vi "Main6.vi"() -> ()   [LabVIEW 2014]
doc: "The myRIO Project template acquires acceleration data from the onboard accelerometer and displays the changes of acceleration values in a waveform chart."
uses:
  <vilib>/myRIO/Instrument Drivers/Onboard IO/AI/typedefs/AI Reference.ctl
  <vilib>/myRIO/Common/Instrument Driver Framework/Utilities/typedefs/myRIO Generic Hardware Reference.ctl
  <vilib>/myRIO/Common/Instrument Driver Framework/Utilities/typedefs/Hardware Version Enum.ctl
  <vilib>/myRIO/Common/Instrument Driver Framework/Utilities/typedefs/myRIO v1.0 Reference.ctl
  <vilib>/myRIO/Common/Instrument Driver Framework/Utilities/typedefs/Generic FPGA Reference.ctl
  <vilib>/myRIO/Common/Instrument Driver Framework/myRIO v1.0/AI/typedefs/AI Channels List.ctl
  <vilib>/myRIO/Common/Instrument Driver Framework/myRIO v1.0/AI/typedefs/AI Channels Enum.ctl
  <vilib>/myRIO/Common/Instrument Driver Framework/Utilities/typedefs/Analog Scaling Constants List.ctl
  <vilib>/myRIO/Common/Instrument Driver Framework/Utilities/typedefs/Analog Scaling Constants.ctl
  <vilib>/userdefined/High Color/nirio_resource_hc.ctl
  <vilib>/myRIO/Instrument Drivers/Onboard IO/DIO/typedefs/DIO Reference.ctl
  <vilib>/myRIO/Common/Instrument Driver Framework/myRIO v1.0/DIO/typedefs/DIO Channels List.ctl
  <vilib>/myRIO/Common/Instrument Driver Framework/myRIO v1.0/DIO/typedefs/DIO Channels Enum.ctl
  <vilib>/myRIO/Common/Instrument Driver Framework/Utilities/vis/Is FPGA Ref Available.vi
  <vilib>/myRIO/Common/Instrument Driver Framework/myRIO v1.0/AI/vis/myRIO v1.1 Open AI.vi
  <vilib>/myRIO/Instrument Drivers/Onboard IO/AI/vis/Read.vi
  <vilib>/myRIO/Common/Instrument Driver Framework/myRIO v1.0/DIO/vis/myRIO v1.1 Open DIO.vi
  <vilib>/myRIO/Instrument Drivers/Onboard IO/DIO/vis/Write.vi
  <vilib>/myRIO/Common/Instrument Driver Framework/Utilities/vis/Validate Channels.vi
  <vilib>/myRIO/Common/Instrument Driver Framework/myRIO v1.0/AI/vis/myRIO v1.0 Reserve AI.vi
  <vilib>/myRIO/Common/Instrument Driver Framework/myRIO v1.0/DIO/vis/myRIO v1.0 Reserve DIO.vi
  <vilib>/myRIO/Common/Instrument Driver Framework/myRIO v1.0/AI/vis/myRIO v1.0 Build MUX Configuration AI.vi
  <vilib>/myRIO/Common/Instrument Driver Framework/myRIO v1.0/Resource Manager/vis/myRIO v1.0 Reserve Channel List.vi
  <vilib>/myRIO/Common/Instrument Driver Framework/myRIO v1.0/DIO/vis/myRIO v1.0 Build MUX Configuration DIO.vi
  <vilib>/myRIO/Common/Instrument Driver Framework/myRIO v1.0/Resource Manager/vis/myRIO v1.0 Reserve Channel.vi
  <vilib>/myRIO/Common/Instrument Driver Framework/myRIO v1.0/Resource Manager/vis/myRIO v1.0 Unreserve Channel.vi
  <vilib>/myRIO/Common/Instrument Driver Framework/myRIO v1.0/Resource Manager/vis/myRIO v1.0 Create Configuration List.vi
  <vilib>/myRIO/Common/Instrument Driver Framework/myRIO v1.0/Resource Manager/vis/myRIO v1.0 Build Mutex Name.vi
  <vilib>/Utility/VariantDataType/GetNumericInfo.vi
  <vilib>/Utility/error.llb/Error Cluster From Error Code.vi
  <vilib>/myRIO/Common/Instrument Driver Framework/myRIO v1.0/myRIO v1.1 Open.vi
  <vilib>/myRIO/Common/Instrument Driver Framework/myRIO v1.0/AI/vis/myRIO v1.0 Get Scaling Constants AI.vi
  <vilib>/myRIO/Common/Instrument Driver Framework/Utilities/vis/IO Manager.vi
  <vilib>/myRIO/Common/Instrument Driver Framework/Utilities/vis/Configuration Manager.vi
  <vilib>/myRIO/Common/Instrument Driver Framework/myRIO v1.0/myRIO v1.0 Close.vi
  <vilib>/myRIO/Common/Instrument Driver Framework/myRIO v1.0/AI/vis/myRIO v1.0 Read AI.vi
  <vilib>/myRIO/Common/Instrument Driver Framework/myRIO v1.0/Resource Manager/vis/myRIO v1.0 Configure IO.vi
  <vilib>/myRIO/Common/Instrument Driver Framework/myRIO v1.0/DIO/vis/myRIO v1.0 Write DIO.vi
  <vilib>/myRIO/Express VI/Onboard IO/AI/AI Express VI.xnode
  <vilib>/myRIO/Instrument Drivers/Onboard IO/AI/vis/myRIO AI Open.xnode
  <vilib>/myRIO/Express VI/Onboard Devices/LED/LED Express VI.xnode
  <vilib>/myRIO/Instrument Drivers/Onboard IO/DIO/vis/myRIO DIO Open.xnode
  <vilib>/vision/driver/NI_Vision_Acquisition_Software.lvlib
  <vilib>/vision/NI_Vision_Development_Module.lvlib
  <vilib>/myRIO/Instrument Drivers/Onboard IO/AI/AI.lvlib
  <vilib>/myRIO/Instrument Drivers/Onboard IO/DIO/DIO.lvlib
panel:
  in  "숫자형":dbl
  in  "탭 컨트롤":enum32{"볼링핀 0", "배경 1", "녹색핀 2"}(tab)
  in  "Blue or Luminance":cluster{i32, i32}(slide)={170, 255} scale=0.0..255.0
  in  "Green or Saturation":cluster{i32, i32}(slide)={0, 90} scale=0.0..255.0
  in  "Red or Hue":cluster{i32, i32}(slide)={0, 255} scale=0.0..255.0
  in  "Blue or Luminance 2":cluster{i32, i32}(slide)={0, 145} scale=0.0..255.0
  in  "Green or Saturation 2":cluster{i32, i32}(slide)={1, 41} scale=0.0..255.0
  in  "Red or Hue 2":cluster{i32, i32}(slide)={0, 255} scale=0.0..255.0
  in  "Blue or Luminance 3":cluster{i32, i32}(slide)={60, 255} scale=0.0..255.0
  in  "Green or Saturation 3":cluster{i32, i32}(slide)={35, 255} scale=0.0..255.0
  in  "Red or Hue 3":cluster{i32, i32}(slide)={50, 130} scale=0.0..255.0
  in  "Select Servo":string(combo)="Servo 1"
  in  "Controller Daisy Chain Position (1 - 4)":u8=1
  out "x <= y?":bool=TRUE
  out "불리언":bool
  out "x/y":dbl=323.5
  out "Acceleration 4":dbl(graph)=1.2646485669999998
  out "x*y":dbl=4.429408028571429
  out "Acceleration 3":dbl(graph)=4.429408028571429
  out "x-y":dbl=-3.5
  in  "y":dbl=20.0
  out "범위내?":bool=TRUE
  out "웨이브폼 차트 2":dbl(graph)=-0.0
  in  "3":u8=3
  in  "Controller 2":u8=2
  in  "Number of Erosion":i32=2
  in  "Threshold Color Mode":enum32{"RGB", "HSL"}(radio)=enum."HSL"
  out "Image 2":T1(plugin-control)
  in  "Stop 2":bool
  out "Image":T1(plugin-control)
  in  "Camera Name":refnum<k21>="cam3" caption="IMAQdx Session"
  # "Control Motor"
  # "Read Encoder"
  # "흰색 : 0/255"
  # "흰색 : 0/90~140"
  # "흰색 : 160~170/255"
  # "흰색 : 0/255"
  # "흰색 : 0/90"
  # "흰색 : 170/255"
  # "녹색 : 50/130"
  # "녹색 : 35/255"
  # "녹색 : 60/255"
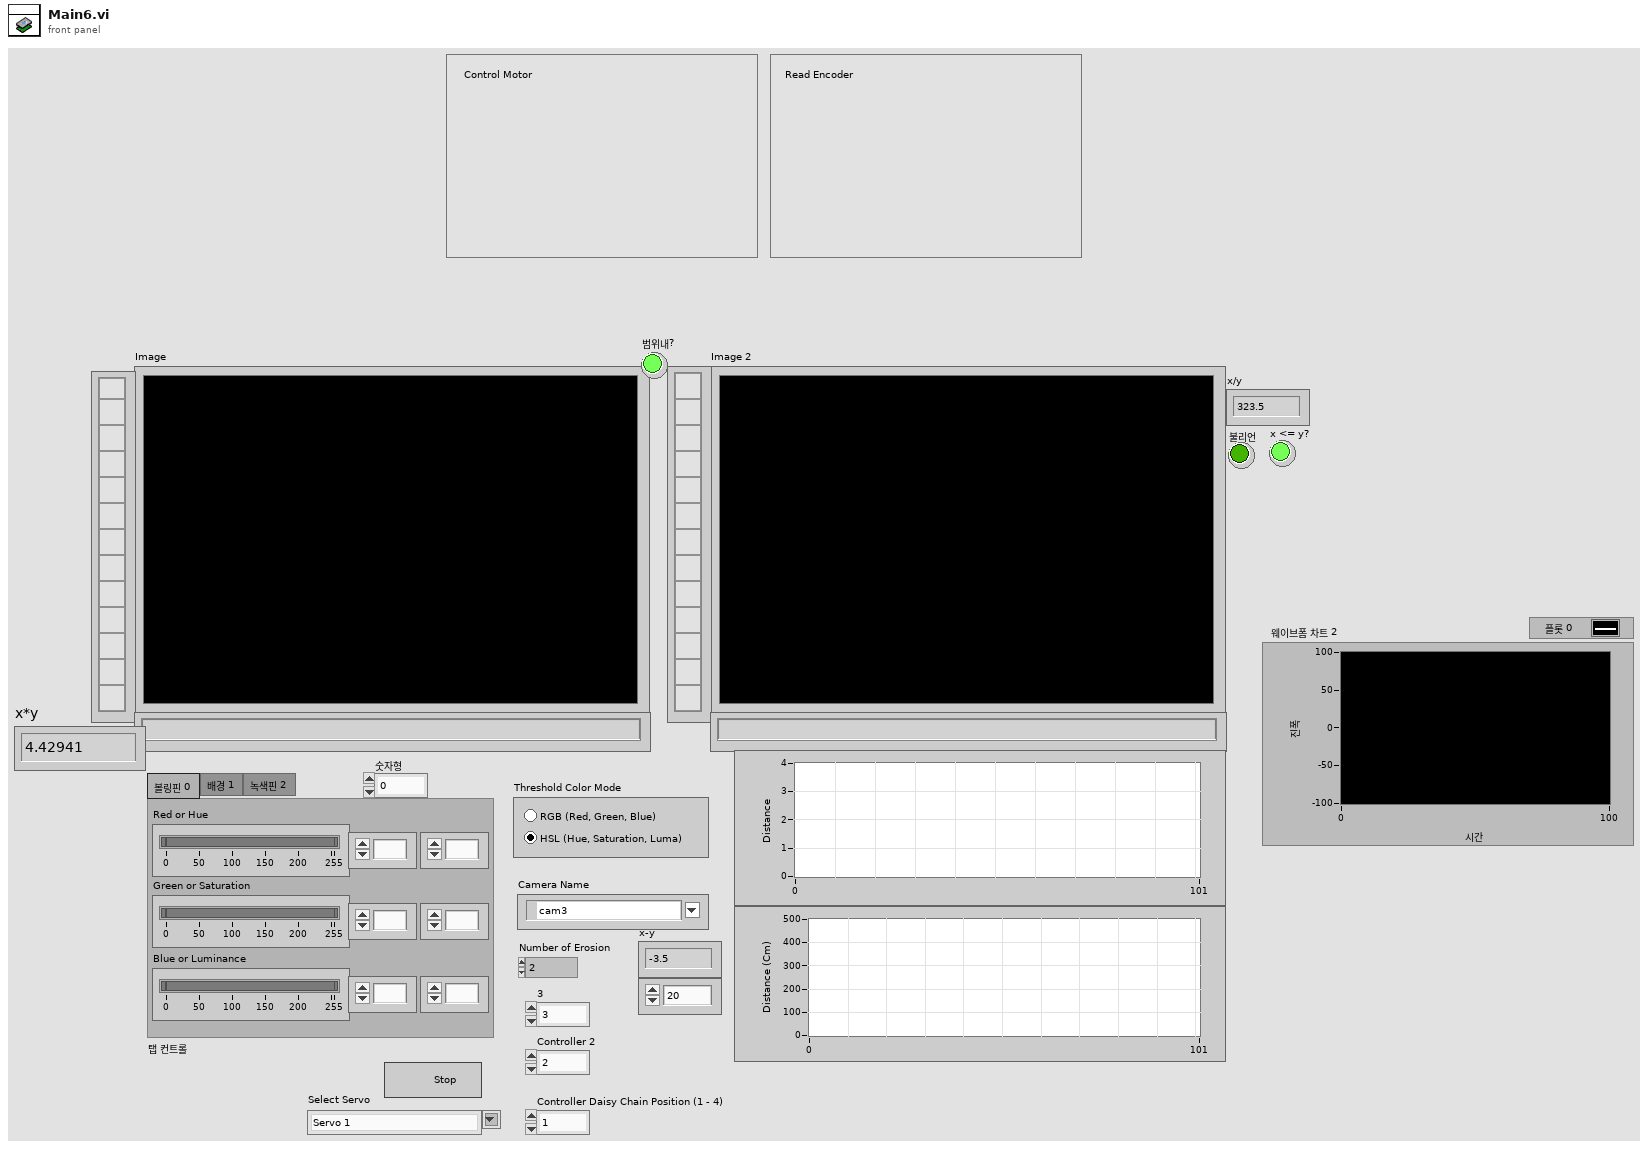
[diagram p1: front panel]
types:
  T1 = typedef "IMAQ Image.ctl" = refnum<image>
  T2 = typedef "DIO.lvlib/DIO Reference.ctl" = cluster{"myRIO Reference":T3, "DIO Channels List":T7}
  T3 = typedef "myRIO Generic Hardware Reference.ctl" = cluster{"myRIO Model":T4, "myRIO Hardware Reference":T5}
  T4 = typedef "Hardware Version Enum.ctl" = enum16{"Unknown", "myRIO-1900", "myRIO-1950"}
  T5 = typedef "myRIO v1.0 Reference.ctl" = cluster{"Generic FPGA Reference":T6, "Allow multiple opens":bool}
  T6 = typedef "Generic FPGA Reference.ctl" = refnum<k20>
  T7 = typedef "DIO Channels List.ctl" = T8[]
  T8 = typedef "DIO Channels Enum.ctl" = enum16{"Not Connected", "C/DIO0", "C/DIO1", "C/DIO2", "C/DIO3", "C/DIO4", "C/DIO5", "C/DIO6", "C/DIO7", "A/DIO0", "A/DIO1", "A/DIO2", "A/DIO3", "A/DIO4", "A/DIO5", "A/DIO6", "A/DIO7", "A/DIO8", "A/DIO9", "A/DIO10", "A/DIO11", "A/DIO12", "A/DIO13", "A/DIO14", "A/DIO15", "B/DIO0", "B/DIO1", "B/DIO2", "B/DIO3", "B/DIO4", "B/DIO5", "B/DIO6", "B/DIO7", "B/DIO8", "B/DIO9", "B/DIO10", "B/DIO11", "B/DIO12", "B/DIO13", "B/DIO14", "B/DIO15", "LED0", "LED1", "LED2", "LED3", "Button0"}
  T9 = typedef "nirio_resource_hc.ctl" = tag
  T10 = typedef "AI.lvlib/AI Reference.ctl" = cluster{"myRIO Reference":T3, "AI Channels List":T11, "AI Scaling Constants List":T13}
  T11 = typedef "AI Channels List.ctl" = T12[]
  T12 = typedef "AI Channels Enum.ctl" = enum16{"Not Connected", "AudioIn/Left", "AudioIn/Right", "C/AI0", "C/AI1", "A/AI0", "A/AI1", "A/AI2", "A/AI3", "B/AI0", "B/AI1", "B/AI2", "B/AI3"}
  T13 = typedef "Analog Scaling Constants List.ctl" = T14[]
  T14 = typedef "Analog Scaling Constants.ctl" = cluster{"LSB Weight (Volts)":dbl, "Offset (Volts)":dbl, "Signed?":bool}
  T15 = typedef "IMAQ Rectangle" = cluster{"Left":i32, "Top":i32, "Right":i32, "Bottom":i32, "Rotation":dbl}
  T16 = typedef "Image Type" = u32
  T17 = typedef "IMAQdx.ctl" = refnum<k21>
  T18 = cluster{"Global Rectangle":i32[], "Contours":cluster{"Contour Type":u32, "ROI Type":u32, "Points":i32[]}[]}
  T19 = cluster{"Area":dbl, "Number of Holes":dbl, "Bounding Rect":cluster{"Left":dbl, "Top":dbl, "Right":dbl, "Bottom":dbl}, "Center of Mass":cluster{"X":dbl, "Y":dbl}, "Orientation":dbl, "Dimensions":cluster{"Width":dbl, "Height":dbl}}[]
  T20 = cluster{"Left":dbl, "Top":dbl, "Right":dbl, "Bottom":dbl}
  T21 = typedef "ROI Descriptor" = cluster{"Global Rectangle":i32[], "Contours":cluster{"ID":enum32{"External", "Internal"}, "Type":u32, "Coordinates":i32[]}[]}
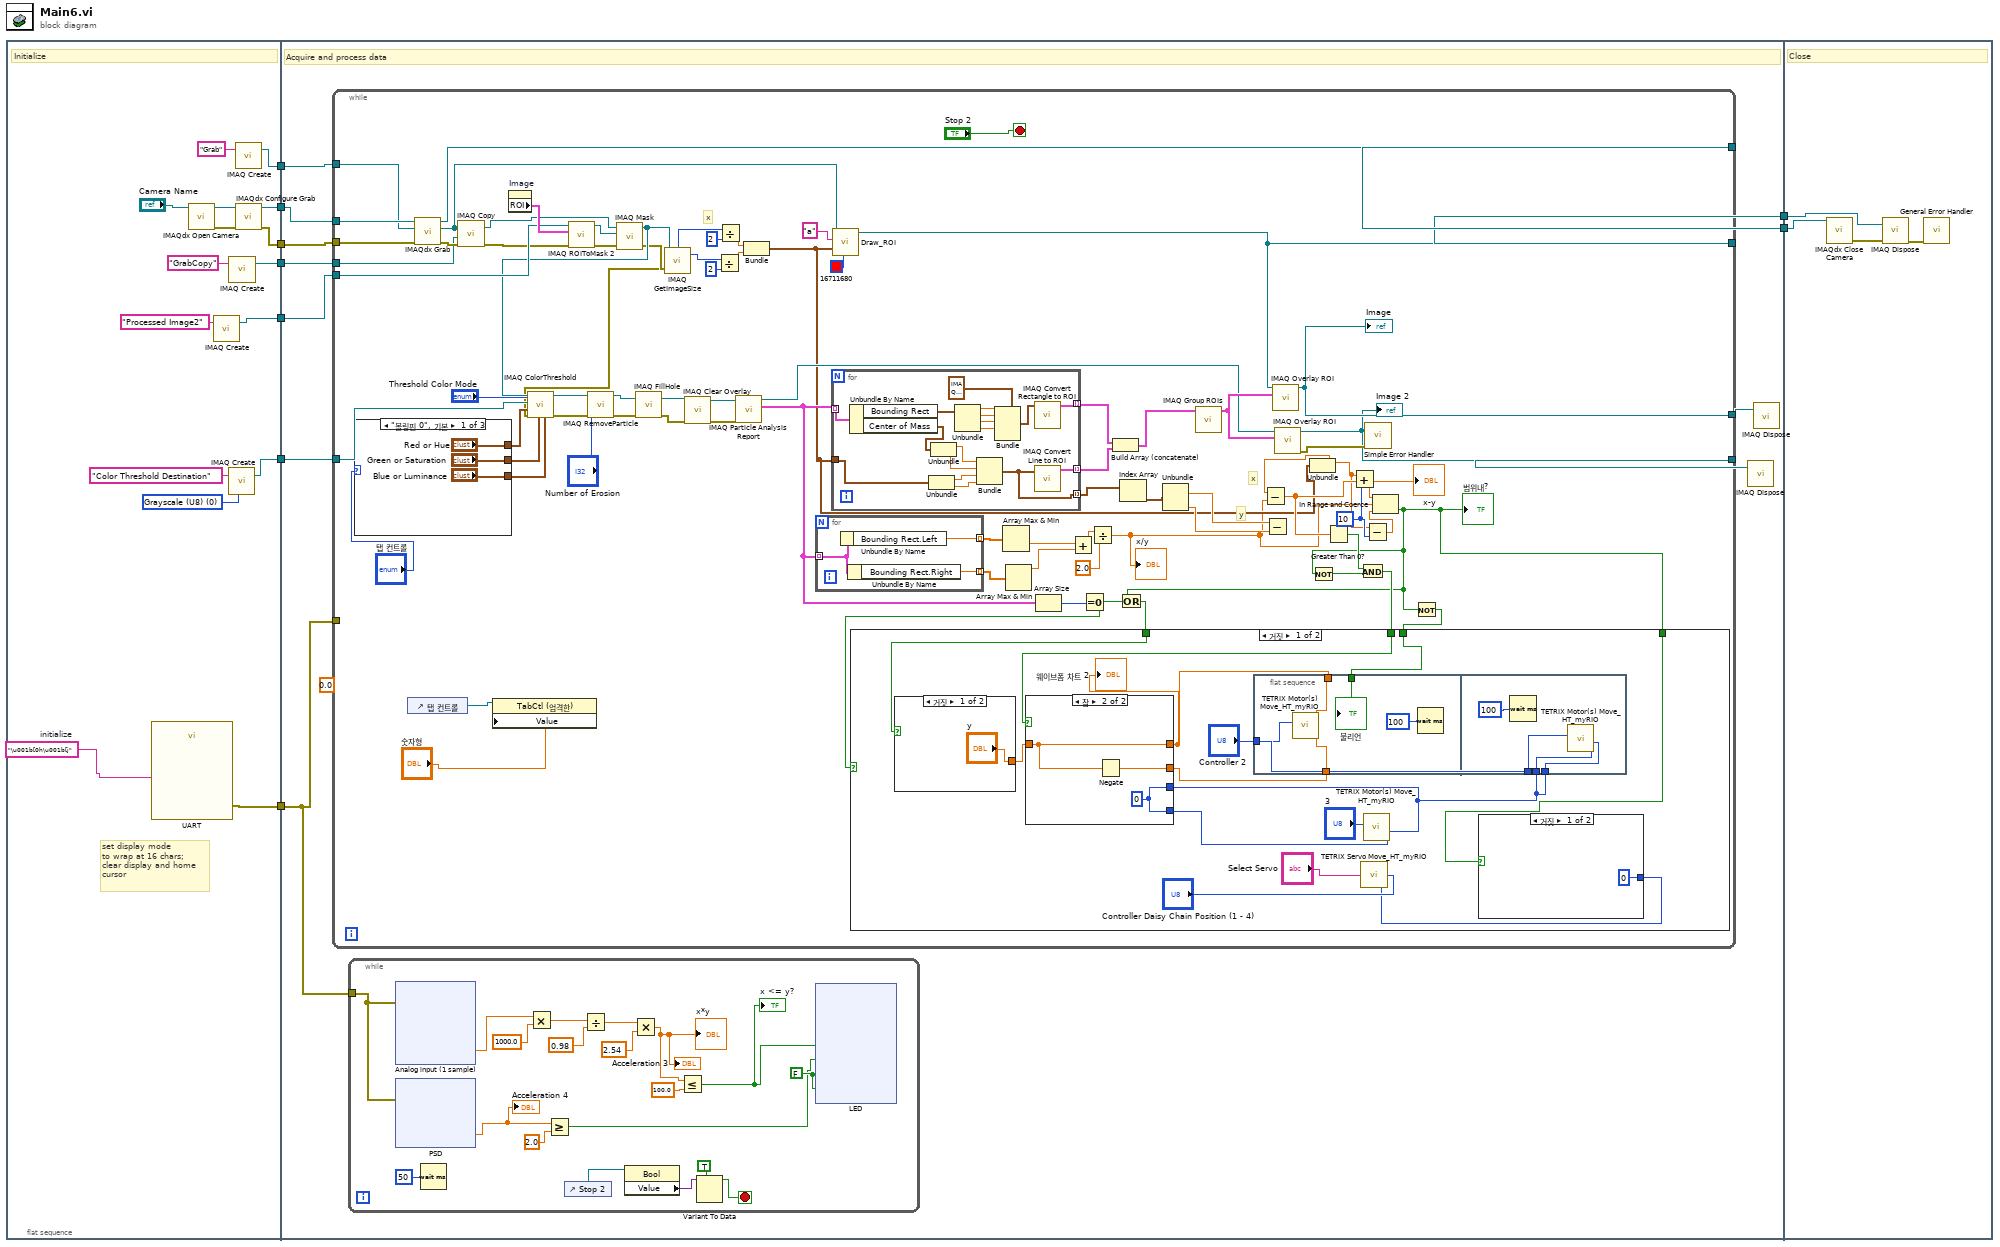
[diagram p0: block diagram]
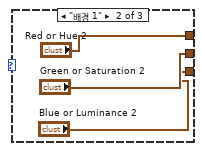
[diagram p2: hidden frame]
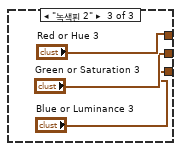
[diagram p3: hidden frame]
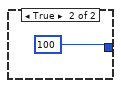
[diagram p4: hidden frame]
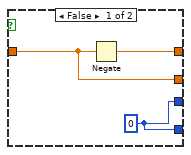
[diagram p5: hidden frame]
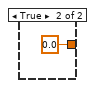
[diagram p6: hidden frame]
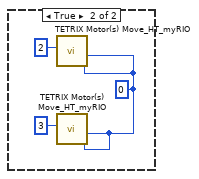
[diagram p7: hidden frame]
diagram:
  n1 = flat-sequence {
    tunnel: [w21] -> w9
    tunnel: [w20] -> w8
    tunnel: [w19] -> w7
    tunnel: [w17] -> w4
    tunnel: [w15] -> w3
    tunnel: [w14] -> w2
    tunnel: [w11] -> w1
    tunnel: w9 -> [w36]
    tunnel: w8 -> [w35]
    tunnel: w7 -> [w34]
    tunnel: [w28] -> w6
    tunnel: [w33] -> w5
    tunnel: w4 -> [w30]
    tunnel: w3 -> [w29]
    tunnel: w2 -> [w26]
    tunnel: w1 -> [w27]
    tunnel: w6 -> [w311]
    tunnel: w5 -> [w310]
    frame #0 {
      w10 = "\u001b[0h\u001b[j"  # initialize
      w13 = T16 0 items=["Grayscale (U8)", "Grayscale (I16)", "Grayscale (SGL)", "Complex (CSG)", "RGB (U32)", "HSL (U32)", "RGB (U64)", "Grayscale (U16)"] ("Image Type")
      # "set display mode\nto wrap at 16 chars;\nclear display and home\ncursor"
      # "Initialize"
      n2 = call "UART"("Characters to Write"=w10) -> ("error out"=w14:errorcluster)  [unwired: 25 in, 1 out]
      n3 = call <vilib>:"IMAQdx Open Camera.vi"("Session In"="Camera Name") -> ("error out"=w25:errorcluster, "Session Out"=w24:T17)  [unwired: 2 in, 7 out]
      n4 = call "IMAQ Create"("Image Name"="Processed Image2") -> ("New Image"=w17:T1)  [unwired: 3 in, 2 out]
      n5 = call "IMAQ Create"("Image Name"="Color Threshold Destination", "Image Type"=w13) -> ("New Image"=w11:T1)  [unwired: 3 in, 1 out]
      n6 = call "IMAQ Create"("Image Name"="GrabCopy") -> ("New Image"=w15:T1)  [unwired: 3 in, 2 out]
      n7 = call "IMAQ Create"("Image Name"="Grab") -> ("New Image"=w21:T1)  [unwired: 3 in, 2 out]
      n8 = call <vilib>:"IMAQdx Configure Grab.vi"("error in"=w25, "Session In"=w24) -> ("error out"=w19:errorcluster, "Session Out"=w20:T17)  [unwired: 8 out]
    }
    frame #1 {
      (unwired) 0.0 ("y")
      # "Acquire and process data"
      n9 = while {
        tunnel: [w241] -> w33
        tunnel: w34 -> [w243]
        tunnel: w35 -> [w244]
        tunnel: w36 -> [w242]
        tunnel: [w213] -> w32
        tunnel: [w212] -> w31
        tunnel: w30 -> [w234]
        tunnel: w29 -> [w220]
        tunnel: [w214] -> w28
        tunnel: w26 -> [_]
        tunnel: w27 -> [w205]
        stop <- "Stop 2" stop-if-true
        w175 = 10
        # "y"
        # "x"
        # "x"
        n10 = case shown="\"볼링핀 0\", 기본" "탭 컨트롤" {
          tunnel: ["Blue or Luminance" "Blue or Luminance 2" "Blue or Luminance 3"] -> w203
          tunnel: ["Red or Hue" "Red or Hue 2" "Red or Hue 3"] -> w202
          tunnel: ["Green or Saturation" "Green or Saturation 2" "Green or Saturation 3"] -> w201
          frame "볼링핀 0", Default {
          }
          frame "배경 1" {
          }
          frame "녹색핀 2" {
          }
        }
        n11 = control-ref of="탭 컨트롤"() -> (w181:refnum<vi>)
        n12 = call <vilib>:"IMAQdx Grab.vi"("error in"=w243, "Image In"=w242, "Session In"=w244) -> ("error out"=w222:errorcluster, "Image Out"=w218:T1, "Session Out"=w241:T17)  [unwired: 1 in, 5 out]
        n13 = call "IMAQ Copy"("error in (no error)"=w222, "Image Dst"=w220, "Image Src"=w218) -> ("error out"=w221:errorcluster, "Image Dst Out"=w219:T1)  [unwired: 3 in]
        n14 = property class="TabCtl (엄격한)"(reference=w181, "Value"="숫자형") -> ()  [unwired: 1 in, 2 out]
        n15 = property on="Image" class="ImageControl"() -> ("ROI"=w236:T18)  [unwired: 2 in, 2 out]
        n16 = call "IMAQ ROIToMask 2"("error in (no error)"=w221, "ROI Descriptor"=w236, "Image"=w234) -> ("error out"=w232:errorcluster, "Image Out"=w233:T1)  [unwired: 6 in, 1 out]
        n17 = call "IMAQ Mask"("error in (no error)"=w232, "Image Mask"=w233, "Image Src"=w219) -> ("error out"=w211:errorcluster, "Image Dst Out"=w217:T1)  [unwired: 2 in]
        n18 = call "IMAQ GetImageSize"("Image"=w217, "error in (no error)"=w211) -> ("Y Resolution"=w227:i32, "X Resolution"=w230:i32, "error out"=w197:errorcluster)  [unwired: 2 in]
        n19 = call "IMAQ ColorThreshold"("Blue or Luma or Val or Inten Range"=w203, "Green or Sat Range"=w201, "Color Mode"="Threshold Color Mode", "error in (no error)"=w197, "Red or Hue Range"=w202, "Image Dst"=w205, "Image Src"=w217) -> ("error out"=w198:errorcluster, "Image Dst Out"=w200:T1)  [unwired: 3 in]
        n20 = call "IMAQ RemoveParticle"("error in (no error)"=w198, "Number of Erosion"="Number of Erosion", "Image Src"=w200) -> ("error out"=w193:errorcluster, "Image Dst Out"=w194:T1)  [unwired: 7 in]
        n21 = call "IMAQ FillHole"("error in (no error)"=w193, "Image Src"=w194) -> ("error out"=w196:errorcluster, "Image Dst Out"=w195:T1)  [unwired: 4 in]
        n22 = call "IMAQ Clear Overlay"("error in (no error)"=w196, "Image"=w195) -> ("error out"=w231:errorcluster, "Image Out"=w238:T1)  [unwired: 1 in, 7 out]
        n23 = Divide(x=w227, y=2) -> (x/y=w225:dbl)
        n24 = Divide(x=w230, y=2) -> (x/y=w226:dbl)
        n25 = call "IMAQ Particle Analysis Report"("error in (no error)"=w231, "Image"=w238) -> ("Particle Reports (Pixels)"=w190:T19, "Image Out (duplicate)"=w237:T1)  [unwired: 4 in, 4 out]
        n26 = Bundle(w226, w225) -> (w178:cluster{dbl, dbl})  [unwired: 1 in]
        n27 = for {
          tunnel: w190 -> [w292] mode=indexing
          tunnel: [w291] -> w172 mode=indexing
          tunnel: [w290] -> w170 mode=indexing
          n28 = Unbundle By Name(w292) -> ("Bounding Rect.Left"=w291:dbl)
          n29 = Unbundle By Name(w292) -> ("Bounding Rect.Right"=w290:dbl)
        }
        n30 = for {
          tunnel: w190 -> [w309] mode=indexing
          tunnel: [w301] -> w216 mode=indexing
          tunnel: w178 -> [w297]
          tunnel: [w294] -> w210 mode=indexing
          tunnel: [w293] -> w209 mode=indexing
          n31 = Unbundle By Name(w309) -> ("Bounding Rect"=w307:T20, "Center of Mass"=w300:cluster{"X":dbl, "Y":dbl})
          n32 = Unbundle(w297) -> (w296:dbl, w295:dbl)
          n33 = Unbundle(w300) -> ("X"=w299:dbl, "Y"=w298:dbl)
          n34 = Unbundle(w307) -> ("Left"=w306:dbl, "Top"=w305:dbl, "Right"=w304:dbl, "Bottom"=w303:dbl)
          n35 = Bundle("X"=w299, "Y"=w298, w296, w295) -> (w293:cluster{"X":dbl, "Y":dbl, dbl, dbl})  [unwired: 1 in]
          n36 = Bundle(cluster=T15 {"Left"=0, "Top"=0, "Right"=0, "Bottom"=0, "Rotation"=0.0} ("Rectangle"), "Left"=w306, "Top"=w305, "Right"=w304, "Bottom"=w303) -> (w302:T15)  [unwired: 1 in]
          n37 = call "IMAQ Convert Rectangle to ROI"("Rectangle"=w302) -> ("ROI Descriptor"=w301:T21)  [unwired: 8 in, 1 out]
          n38 = call "IMAQ Convert Line to ROI"("Line"=w293) -> ("ROI Descriptor"=w294:T21)  [unwired: 8 in, 1 out]
        }
        n39 = call "Draw_ROI.vi"("Color"=u32 16711680, "클러스터"=w178, "Group"="a", "참조 번호 입력"=w218) -> ("참조 번호 출력"=w214:T1)  [unwired: 7 in]
        n40 = Array Max & Min(array=w172) -> (min value=w171:dbl)  [unwired: 3 out]
        n41 = Array Max & Min(array=w170) -> (max value=w169:dbl)  [unwired: 3 out]
        n42 = Array Size(array=w190) -> (size(s)=w184:i32)
        n43 = Add(x=w171, y=w169) -> (x+y=w189:dbl)
        n44 = Equal To 0?(x=w184) -> (x = 0?=w183:bool)
        n45 = Divide(x=w189, y=2.0) -> (x/y=w173:dbl)
        "x/y" <- w173
        n46 = Build Array (concatenate)(w216, w210) -> (w215:T21[])
        n47 = Index Array(array=w209) -> (element=w208:cluster{"X":dbl, "Y":dbl, dbl, dbl})  [unwired: 1 in]
        n48 = Unbundle(w208) -> ("Y"=w207:dbl, w206:dbl)  [unwired: 2 out]
        n49 = call "IMAQ Group ROIs"("ROI Descriptors"=w215) -> ("ROI Descriptor out"=w239:T21)  [unwired: 1 in, 3 out]
        n50 = Subtract(x=w207, y=w206) -> ()  [unwired: 1 out]
        n51 = call "IMAQ Overlay ROI"("ROI Descriptor"=w239, "Image"=w214) -> ("Image Out"=w213:T1)  [unwired: 4 in, 5 out]
        "Image" <- w213
        n52 = call "IMAQ Overlay ROI"("ROI Descriptor"=w239, "Image"=w237) -> ("error out"=w240:errorcluster, "Image Out"=w212:T1)  [unwired: 4 in, 4 out]
        "Image 2" <- w212
        n53 = Unbundle(w178) -> (w174:dbl)  [unwired: 1 out]
        n54 = Subtract(x=w174, y=w173) -> (x-y=w187:dbl)
        "x-y" <- w187
        n55 = Greater Than 0?(x=w187) -> (x > 0?=w192:bool)
        n56 = Add(x=w174, y=w175) -> (x+y=w177:dbl)
        n57 = Subtract(x=w174, y=w175) -> (x-y=w176:dbl)
        n58 = call <vilib>:"Simple Error Handler.vi"("error in (no error)"=w240) -> ()  [unwired: 1 in, 8 out]
        n59 = In Range and Coerce(upper limit=w177, x=w173, lower limit=w176) -> (In Range?=w168:bool)  [unwired: 1 out]
        "범위내?" <- w168
        n60 = Or(x=w168, y=w183) -> (x .or. y?=w185:bool)
        n61 = Not(x=w168) -> (.not. x?=w191:bool)
        n62 = And(x=w192, y=w191) -> (x .and. y?=w186:bool)
        n63 = Not(x=w168) -> (.not. x?=w179:bool)
        n64 = case shown="거짓" w183 {
          tunnel: w186 -> [w259 _]
          tunnel: w185 -> [w258 _]
          tunnel: w179 -> [w257 _]
          tunnel: w168 -> [w256 _]
          frame False {
            n65 = case shown="거짓" w258 {
              tunnel: ["y" 0.0 ("y")] -> w266
              frame False {
              }
              frame True {
              }
            }
            n66 = case shown="참" w259 {
              tunnel: [w281 w284] -> w265
              tunnel: w266 -> [w280 w284]
              tunnel: [w280 w283] -> w264
              tunnel: [w279 w282] -> w263
              tunnel: [w279 w282] -> w261
              frame False {
                w279 = 0
                n67 = Negate(x=w280) -> (-x=w281:dbl)
              }
              frame True {
                w282 = 0
                n68 = Negate(x=w284) -> (-x=w283:dbl)
              }
            }
            "웨이브폼 차트 2" <- w265
            n69 = flat-sequence {
              tunnel: "Controller 2" -> [w274]
              tunnel: w265 -> [w273]
              tunnel: w264 -> [w272]
              tunnel: w257 -> [w270]
              tunnel: "Controller 2" -> [w278]
              tunnel: w261 -> [w277]
              tunnel: w261 -> [w276]
              frame #0 {
                n70 = call <vilib>:"TETRIX Motor(s) Move_HT_myRIO.vi"("Motor 2 Power (-100 to 100)\n0 = Stop/Brake\n-128 = Stop/Coast"=w272, "Motor 1 Power (-100 to 100)\n0 = Stop/Brake\n-128 = Stop/Coast"=w273, "Controller Daisy Chain Position: 1 - 4"=w274) -> ()  [unwired: 6 in, 1 out]
                n71 = Wait (ms)(milliseconds to wait=u32 100 ("대기 시간(ms)")) -> ()  [unwired: 1 out]
                "불리언" <- w270
              }
              frame #1 {
                n72 = Wait (ms)(milliseconds to wait=u32 100 ("대기 시간(ms)")) -> ()  [unwired: 1 out]
                n73 = call <vilib>:"TETRIX Motor(s) Move_HT_myRIO.vi"("Motor 2 Power (-100 to 100)\n0 = Stop/Brake\n-128 = Stop/Coast"=w277, "Motor 1 Power (-100 to 100)\n0 = Stop/Brake\n-128 = Stop/Coast"=w276, "Controller Daisy Chain Position: 1 - 4"=w278) -> ()  [unwired: 6 in, 1 out]
              }
            }
            n74 = call <vilib>:"TETRIX Motor(s) Move_HT_myRIO.vi"("Motor 2 Power (-100 to 100)\n0 = Stop/Brake\n-128 = Stop/Coast"=w263, "Motor 1 Power (-100 to 100)\n0 = Stop/Brake\n-128 = Stop/Coast"=w261, "Controller Daisy Chain Position: 1 - 4"="3") -> ()  [unwired: 6 in, 1 out]
            n75 = case shown="거짓" w256 {
              tunnel: [u8 0 ("Controller Daisy Chain Position (1 - 4)") u8 100 ("Controller Daisy Chain Position (1 - 4)")] -> w254
              frame False {
              }
              frame True {
              }
            }
            n76 = call <vilib>:"TETRIX Servo Move_HT_myRIO.vi"("Servo Position (0 - 255)"=w254, "Controller Daisy Chain Position (1 - 4)"="Controller Daisy Chain Position (1 - 4)", "Select Servo"="Select Servo") -> ()  [unwired: 2 in, 1 out]
          }
          frame True {
            w287 = 0
            n77 = call <vilib>:"TETRIX Motor(s) Move_HT_myRIO.vi"("Motor 2 Power (-100 to 100)\n0 = Stop/Brake\n-128 = Stop/Coast"=w287, "Motor 1 Power (-100 to 100)\n0 = Stop/Brake\n-128 = Stop/Coast"=w287, "Controller Daisy Chain Position: 1 - 4"=u8 2) -> ()  [unwired: 6 in, 1 out]
            n78 = call <vilib>:"TETRIX Motor(s) Move_HT_myRIO.vi"("Motor 2 Power (-100 to 100)\n0 = Stop/Brake\n-128 = Stop/Coast"=w287, "Motor 1 Power (-100 to 100)\n0 = Stop/Brake\n-128 = Stop/Coast"=w287, "Controller Daisy Chain Position: 1 - 4"=u8 3) -> ()  [unwired: 6 in, 1 out]
          }
        }
      }
      n79 = while {
        tunnel: w26 -> [w44]
        stop <- w52 stop-if-true
        w41 = FALSE ("LED1")
        n80 = xnode "Analog input (1 sample)"("error in (no error)"=w44) -> ("UltraSonic (A/AI0 (Pin 3))"=w46:dbl)  [unwired: 1 out]
        n81 = xnode "PSD"("error in (no error)"=w44) -> ("C/AI0 (C/AI0 (AI0))"=w38:dbl)  [unwired: 1 out]
        "Acceleration 4" <- w38
        n82 = Wait (ms)(milliseconds to wait=u32 50 ("대기 시간(ms)")) -> ()  [unwired: 1 out]
        n83 = Multiply(x=w46, y=1000.0) -> (x*y=w49:dbl)
        n84 = Greater Or Equal?(x=w38, y=2.0) -> (x >= y?=w37:bool)
        n85 = control-ref of="Stop 2"() -> (w55:refnum<vi>)
        n86 = Divide(x=w49, y=0.98) -> (x/y=w47:dbl)
        n87 = property class="Bool"(reference=w55) -> ("Value"=w54:variant)  [unwired: 1 in, 2 out]
        n88 = Multiply(x=w47, y=2.54) -> (x*y=w43:dbl)
        "x*y" <- w43
        "Acceleration 3" <- w43
        n89 = Less Or Equal?(x=w43, y=100.0) -> (x <= y?=w40:bool)
        "x <= y?" <- w40
        n90 = Variant To Data(type=TRUE, Variant=w54) -> (data=w52:bool)  [unwired: 1 in, 1 out]
        n91 = xnode "LED"("LED0"=w40, "LED1"=w37, "LED2"=w41, "LED3"=w41) -> ()  [unwired: 1 in, 1 out]
      }
      n92 = call "IMAQ Dispose"("Image"=w31) -> ()  [unwired: 5 in, 1 out]
      n93 = call "IMAQ Dispose"("Image"=w32) -> ()  [unwired: 5 in, 1 out]
    }
    frame #2 {
      # "Close"
      n94 = call <vilib>:"IMAQdx Close Camera.vi"("Session In"=w310) -> ("error out"=w313:errorcluster)  [unwired: 1 in, 9 out]
      n95 = call "IMAQ Dispose"("Image"=w311, "error in (no error)"=w313) -> ("error out"=w312:errorcluster)  [unwired: 4 in]
      n96 = call <vilib>:"General Error Handler.vi"("error in (no error)"=w312) -> ()  [unwired: 2 in, 13 out]
    }
  }
